vi "UseFirstDevice.vi"(0 "object in":refnum<class "AD2_WFG_SDK.lvclass">, 5 "error in (no error)":errorcluster) -> (14 "object out":refnum<class "AD2_WFG_SDK.lvclass">, 19 "error out":errorcluster)   [LabVIEW 2019]
uses:
  <userlib>/Olasdwf/Olasdwf.lvlib
  Users/olaja/Desktop/LabForms2.0/LabFormsLvProj/digilent/digilent.lvlib
  AD2_WFG_SDK.lvclass
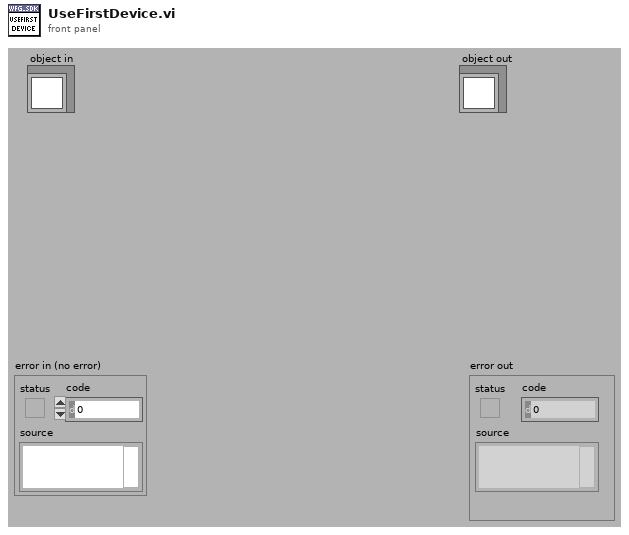
[diagram p1: front panel]
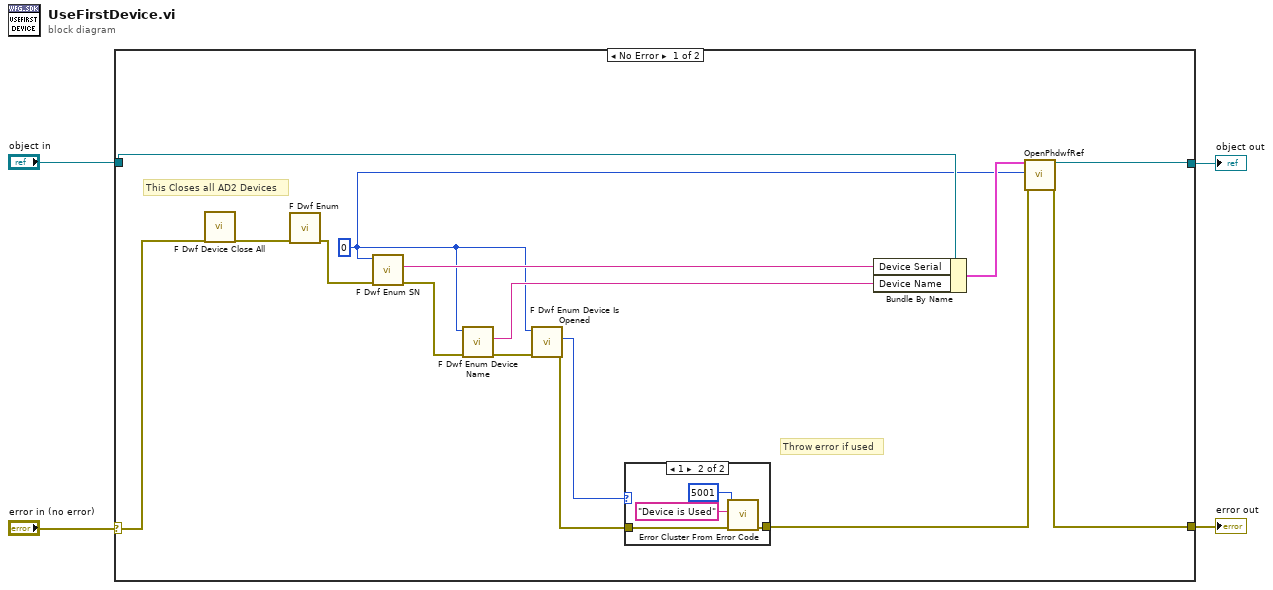
[diagram p0: block diagram]
diagram:
  n1 = case shown="No Error" "error in (no error)" {
    selector: "error in (no error)" -> [w6 w26]
    tunnel: [w8 w26] -> w3
    tunnel: [w10 w25] -> w1
    tunnel: "object in" -> [w19 w25]
    frame No Error {
      w7 = 0 ("idxDevice")
      # "This Closes all AD2 Devices"
      # "Throw error if used"
      n2 = call <userlib>:"F Dwf Device Close All.vi"("error in (no error)"=w6) -> ("error out"=w5:errorcluster)  [unwired: 9 in, 1 out]
      n3 = call <userlib>:"F Dwf Enum.vi"("error in (no error)"=w5) -> ("error out"=w18:errorcluster)  [unwired: 8 in, 2 out]
      n4 = call <userlib>:"F Dwf Enum SN.vi"("error in (no error)"=w18, "idxDevice"=w7) -> ("error out"=w17:errorcluster, "szSN out"=w16:string)  [unwired: 7 in, 1 out]
      n5 = call <userlib>:"F Dwf Enum Device Name.vi"("error in (no error)"=w17, "idxDevice"=w7) -> ("error out"=w12:errorcluster, "szDeviceName out"=w15:string)  [unwired: 7 in, 1 out]
      n6 = call "F Dwf Enum Device Is Opened.vi"("error in (no error)"=w12, "idxDevice"=w7) -> ("error out"=w13:errorcluster, "pfIsUsed out"=w14:i32)  [unwired: 7 in, 1 out]
      n7 = case shown="1" w14 {
        tunnel: w13 -> [w20 w23]
        tunnel: [w20 w22] -> w9
        frame 0, Default {
        }
        frame 1 {
          n8 = call <vilib>:"Error Cluster From Error Code.vi"("error in (no error)"=w23, "error message (\"\")"="Device is Used" ("error message (\"\")"), "error code (0)"=5001) -> ("error out"=w22:errorcluster)  [unwired: 6 in]
        }
      }
      n9 = Bundle By Name(cluster=w19, "Device Serial"=w16, "Device Name"=w15) -> (w11:cluster{})
      n10 = call-dynamic "OpenPhdwfRef.vi"("object in"=w11, "idxDevice"=w7, "error in (no error)"=w9) -> ("object out"=w10:refnum<class "AD2_WFG_SDK.lvclass">, "error out"=w8:errorcluster)  [unwired: 15 in]
    }
    frame Error {
    }
  }
  "error out" <- w3
  "object out" <- w1
